vi "fix exec settings.vi"(8 "error in":errorcluster, 10 "decideprojectfeatures in":refnum<class "DecideModuleFeatures.lvclass">, 11 "user project in":refnum<vi>) -> (0 "error out":errorcluster, 3 "user project out":refnum<vi>)   [LabVIEW 2013, in "DecideModuleFeatures.lvclass"]
uses:
  DecideModuleFeatures.lvclass
  DecideModuleFeatures.lvclass/DecideModuleFeatures.ctl
  Read input_.vi
  Read output_.vi
  Read process_.vi
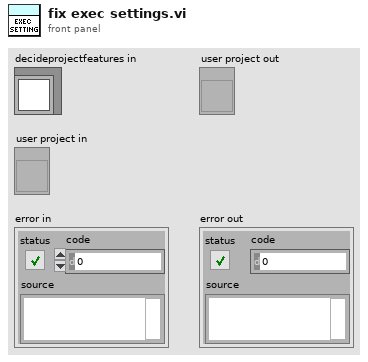
[diagram p1: front panel]
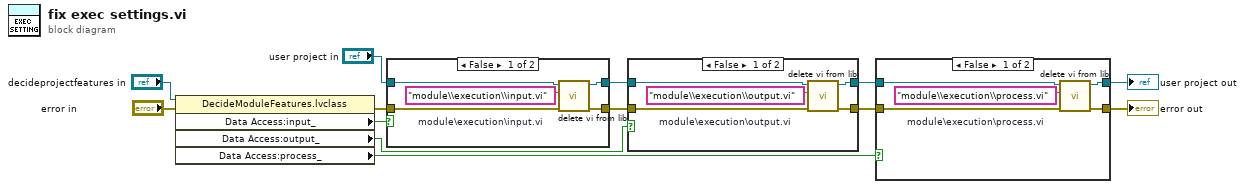
[diagram p0: block diagram]
diagram:
  n1 = property class="DecideModuleFeatures.lvclass"(reference="decideprojectfeatures in", error in="error in") -> (error out=w4:errorcluster, "Data Access:input_"=w3:bool, "Data Access:output_"=w2:bool, "Data Access:process_"=w1:bool)  [unwired: 1 out]
  n2 = case shown="False" w3 {
    tunnel: "user project in" -> [w18 w20]
    tunnel: [w17 w20] -> w10
    tunnel: [w16 w19] -> w5
    tunnel: w4 -> [w15 w19]
    frame False {
      w14 = "module\\execution\\input.vi"  # module\execution\input.vi
      n3 = call "delete vi from lib.vi"("error in"=w15, "relative path"=w14, "project in"=w18) -> ("error out"=w16:errorcluster, "project out"=w17:refnum<vi>)  [unwired: 6 in, 1 out]
    }
    frame True {
    }
  }
  n4 = case shown="False" w2 {
    tunnel: w10 -> [w25 w27]
    tunnel: [w24 w27] -> w9
    tunnel: [w23 w26] -> w6
    tunnel: w5 -> [w22 w26]
    frame False {
      w21 = "module\\execution\\output.vi"  # module\execution\output.vi
      n5 = call "delete vi from lib.vi"("error in"=w22, "relative path"=w21, "project in"=w25) -> ("error out"=w23:errorcluster, "project out"=w24:refnum<vi>)  [unwired: 6 in, 1 out]
    }
    frame True {
    }
  }
  n6 = case shown="False" w1 {
    tunnel: w9 -> [w32 w34]
    tunnel: [w31 w34] -> w8
    tunnel: [w30 w33] -> w7
    tunnel: w6 -> [w29 w33]
    frame False {
      w28 = "module\\execution\\process.vi"  # module\execution\process.vi
      n7 = call "delete vi from lib.vi"("error in"=w29, "relative path"=w28, "project in"=w32) -> ("error out"=w30:errorcluster, "project out"=w31:refnum<vi>)  [unwired: 6 in, 1 out]
    }
    frame True {
    }
  }
  "error out" <- w7
  "user project out" <- w8
